vi "SAOMM-FormatSet.vi"() -> ()   [LabVIEW 2011]
panel:
  in  "ACK Refnum":refnum<vi>
  in  "Value (little endianed byte array)":u8[](array[numeric])
  in  "Active SET":string
  in  "Command-Array":cluster{"Command":string, "TypeEnum":u32}[](array[cluster])
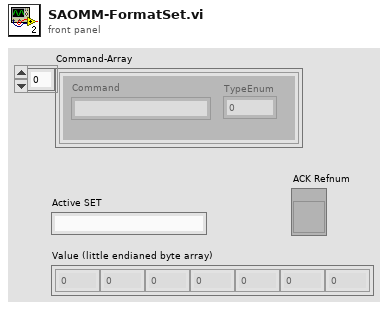
[diagram p1: front panel]
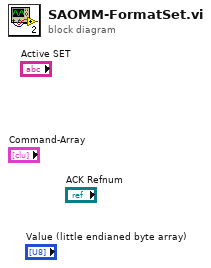
[diagram p0: block diagram]
diagram:
